vi "CustomPID_v3.0.vi"(0 "Kp":dbl=3e-05, 1 "Process Variable":dbl, 2 "Goal":dbl, 5 "Ki":dbl=5e-06, 7 "Kd":dbl=1e-06, 9 "N-Diff":i32=50, 11 "N-Int":i32=50, 12 "Reinit":bool, 13 "Max Ouput":dbl=1.0, 14 "Min Output":dbl=-1.0) -> (4 "Current Error":dbl, 8 "Command":dbl, 10 "Contribution Tracking":cluster{dbl, dbl, dbl}(graph), 15 "PID Tracking":cluster{"Goal Wheel Position":dbl, dbl}(graph)={"Goal Wheel Position"=0.0, -90.17571233858979})   [LabVIEW 2018]
uses:
  <vilib>/Analysis/NI_AALPro.lvlib
panel:
  out "Absolute Iterations":i32
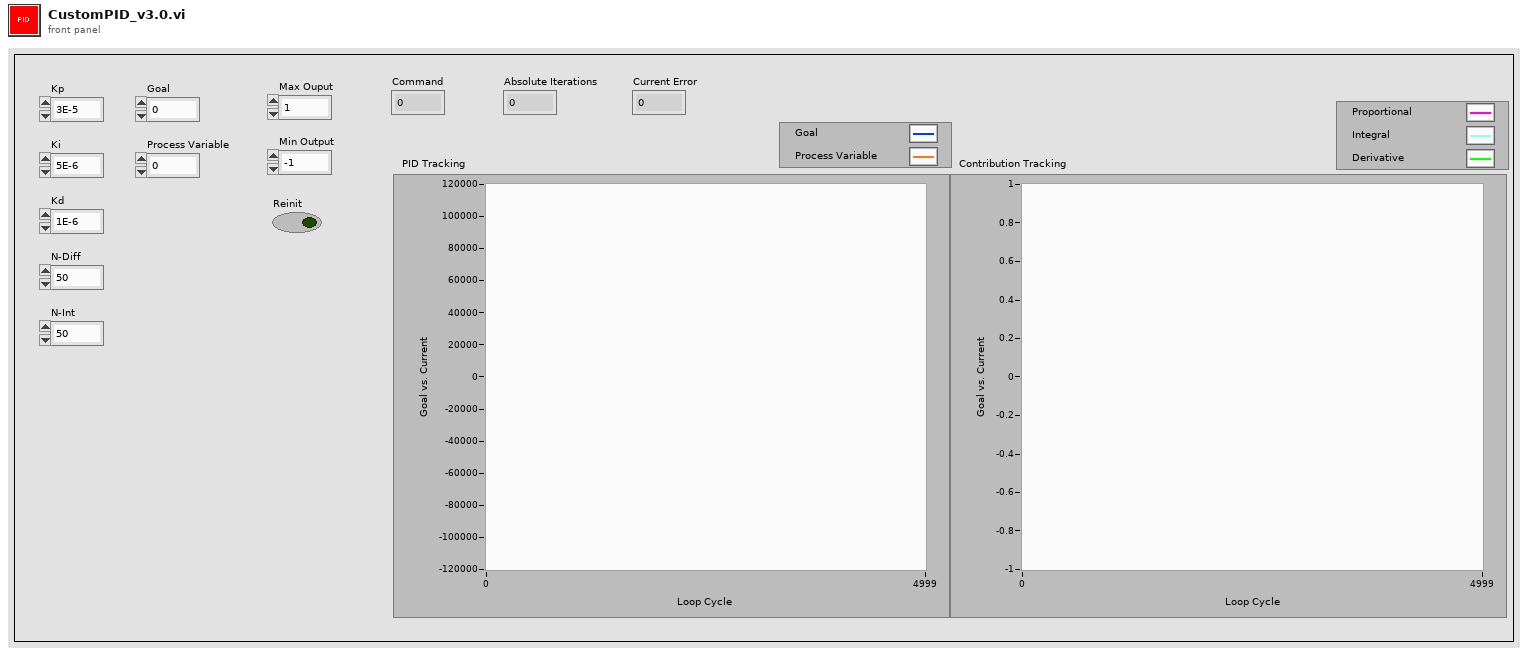
[diagram p1: front panel]
types:
  T1 = cluster{"Max Ouput":dbl, "Max Ouput":dbl, "Max Ouput":dbl}
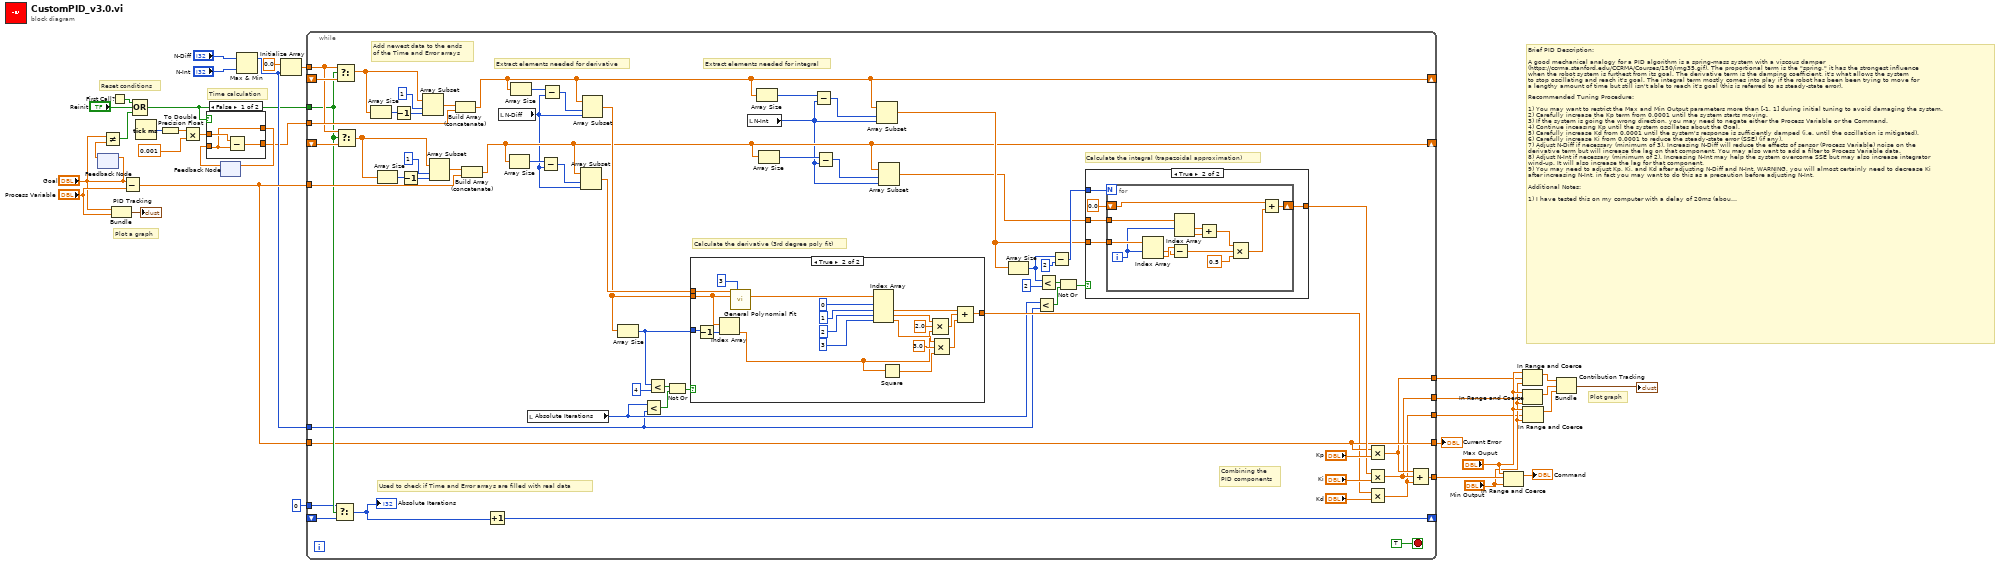
[diagram p0: block diagram]
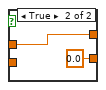
[diagram p2: hidden frame]
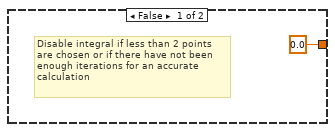
[diagram p3: hidden frame]
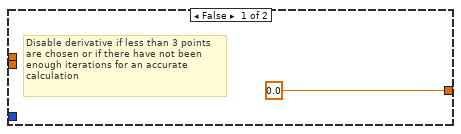
[diagram p4: hidden frame]
diagram:
  # "Plot graph"
  # "Time calculation"
  # "Brief PID Description:\n\nA good mechanical analogy for a PID algorithm is a spring-mass system with a viscous damper \n(https://ccrma.stanford.edu/CCRMA/Courses/150/img35.gif). The proportional term is the \"spring,\" it has the strongest influence\nwhen the robot system is furthest from its goal. The derivative term is the damping coefficient, it's what allows the system\nto stop oscillating and reach it's goal. The integral term mostly comes into play if the robot has been been trying to move for \na lengthy amount of time but still isn't able to reach it's goal (this is referred to as steady-state error).\n\nRecommended Tuning Procedure:\n\n1) You may want to restrict the Max and Min Output parameters more than [-1, 1] during initial tuning to avoid damaging the system.\n2) Carefully increase the Kp term from 0.0001 until the system starts moving.\n3) If the system is going the wrong direction, you may need to negate either the Process Variable or the Command.\n4) Continue inceasing Kp until the system oscillates about the Goal.\n5) Carefully increase Kd from 0.0001 until the system's response is sufficiently damped (i.e. until the oscillation is mitigated).\n6) Carefully increase Ki from 0.0001 to reduce the steady-state error (SSE) (if any).\n7) Adjust N-Diff if necessary (minimum of 3). Increasing N-Diff will reduce the effects of sensor (Process Variable) noise on the \nderivative term but will increase the lag on that component. You may also want to add a filter to Process Variable data.\n8) Adjust N-Int if necessary (minimum of 2). Increasing N-Int may help the system overcome SSE but may also increase integrator\nwind-up. It will also increase the lag for that component.\n9) You may need to adjust Kp, Ki, and Kd after adjusting N-Diff and N-Int. WARNING, you will almost certainly need to decrease Ki\nafter increasing N-Int, in fact you may want to do this as a precaution before adjusting N-Int. \n\nAdditional Notes:\n\n1) I have tested this on my computer with a delay of 20ms (about what I expect for the robot) and it appears to function correctly.\nThat being said I have NOT tested this on an actual, physical system. So exercise caution when testing it for the first time.\n2) Make sure that execution type for all instances of this VI are set to \"preallocated clone reentrant execution.\"\n3) Several parts of this VI were inspired by a PID algorithm written by Dr. Ira Hill at the University of Florida.\n4) If you have any questions, feel free to contact me at lrscime@ufl.edu."
  # "Plot a graph"
  # "Reset conditions"
  n1 = feedback-in #1("Goal") -> ()
  n2 = feedback #1() -> (w21:dbl)  [unwired: 1 in]
  n3 = Not Equal?(x="Goal", y=w21) -> (x != y?=w20:bool)
  n4 = First Call?() -> (First Call?: T/F=w29:bool)
  n5 = Bundle("Goal"="Goal", "Process Variable"="Process Variable") -> (→"PID Tracking":cluster{"Goal":dbl, "Process Variable":dbl})  [unwired: 1 in]
  n6 = Subtract(x="Goal", y="Process Variable") -> (x-y=w34:dbl)
  n7 = Compound Arithmetic op=OR(w29, "Reinit", w20) -> (w11:bool)
  n8 = Tick Count (ms)() -> (millisecond timer value=w18:u32)
  n9 = To Double Precision Float(number=w18) -> (double precision float=w17:dbl)
  n10 = Multiply(x=w17, y=0.001) -> (x*y=w15:dbl)
  n11 = feedback #2() -> (w13:dbl)  [unwired: 1 in]
  n12 = case shown="False" w11 {
    tunnel: w15 -> [w37 w39]
    tunnel: [w35 w39] -> w14
    tunnel: [w36 0.0] -> w12
    tunnel: w13 -> [w35 _]
    frame False {
      n13 = Subtract(x=w37, y=w35) -> (x-y=w36:dbl)
    }
    frame True {
    }
  }
  n14 = feedback-in #2(w14) -> ()
  n15 = Max & Min(x="N-Diff", y="N-Int") -> (max(x,y)=w23:i32)  [unwired: 1 out]
  n16 = Initialize Array(0.0 ("element"), w23) -> (w25:dbl[])
  n17 = while {
    tunnel: [w96] -> w31
    tunnel: w34 -> [w87]
    shift-right: [w75] -> _
    shift-left: _ -> [w61]
    tunnel: w12 -> [w91]
    shift-right: [w62] -> _
    shift-left: _ -> [w58]
    tunnel: w23 -> [w44]
    tunnel: w34 -> [w49]
    shift-right: [w68] -> _
    shift-left: _ -> [w55]
    tunnel: w11 -> [w54]
    tunnel: w25 -> [w59]
    tunnel: 0 -> [w50]
    tunnel: [w49] -> w10
    tunnel: [w42] -> w3
    tunnel: [w41] -> w2
    tunnel: [w40] -> w1
    stop <- TRUE stop-if-true
    # "Combining the\nPID components"
    # "Add newest data to the ends\nof the Time and Error arrays"
    # "Used to check if Time and Error arrays are filled with real data"
    # "Extract elements needed for integral"
    # "Extract elements needed for derivative"
    # "Calculate the integral (trapezoidal approximation)"
    # "Calculate the derivative (3rd degree poly fit)"
    n18 = Select(t=w50, s=w54, f=w55) -> (s? t:f=w56:i32)
    "Absolute Iterations" <- w56
    n19 = Select(t=w59, s=w54, f=w61) -> (s? t:f=w60:dbl[])
    n20 = Select(t=w59, s=w54, f=w58) -> (s? t:f=w57:dbl[])
    n21 = Array Size(array=w60) -> (size(s)=w94:i32)
    n22 = Array Size(array=w57) -> (size(s)=w89:i32)
    n23 = Decrement(x=w94) -> (x-1=w93:i32)
    n24 = Decrement(x=w89) -> (x-1=w88:i32)
    n25 = Array Subset(array=w60, index=1, length=w93) -> (w92:dbl[])
    n26 = Array Subset(array=w57, index=1, length=w88) -> (w86:dbl[])
    n27 = Build Array (concatenate)(w92, w91) -> (w75:dbl[])
    n28 = Build Array (concatenate)(w86, w87) -> (w62:dbl[])
    n29 = Increment(x=w56) -> (x+1=w68:i32)
    n30 = local read "N-Diff"() -> (w52:i32)
    n31 = Array Size(array=w62) -> (size(s)=w82:i32)
    n32 = Array Size(array=w75) -> (size(s)=w85:i32)
    n33 = local read "Absolute Iterations"() -> (w45:i32)
    n34 = Subtract(x=w82, y=w52) -> (x-y=w83:i32)
    n35 = Subtract(x=w85, y=w52) -> (x-y=w84:i32)
    n36 = Array Subset(array=w62, index=w83, length=w52) -> (w81:dbl[])
    n37 = Array Subset(array=w75, index=w84, length=w52) -> (w80:dbl[])
    n38 = Array Size(array=w80) -> (size(s)=w79:i32)
    n39 = Less?(x=w45, y=w44) -> (x < y?=w43:bool)
    n40 = Less?(x=w79, y=4) -> (x < y?=w47:bool)
    n41 = Not Or(1:w43, 2:w47) -> (0:w46:bool)
    n42 = case shown="True" w46 {
      tunnel: w81 -> [_ w136]
      tunnel: w79 -> [_ w135]
      tunnel: w80 -> [_ w133]
      tunnel: [0.0 w129] -> w48
      frame False {
        # "Disable derivative if less than 3 points \nare chosen or if there have not been \nenough iterations for an accurate \ncalculation"
      }
      frame True {
        n43 = Decrement(x=w135) -> (x-1=w134:i32)
        n44 = Index Array(array=w133, index=w134) -> (element=w122:dbl)
        n45 = call <vilib>:"General Polynomial Fit.vi"("Y"=w136, "polynomial order"=3, "X"=w133) -> ("Polynomial Coefficients"=w139:dbl[])  [unwired: 9 in, 3 out]
        n46 = Index Array(array=w139, index #1=0 ("index"), index #2=1 ("index"), index #3=2 ("index"), index #4=3 ("index")) -> (element #2=w128:dbl, element #3=w126:dbl, element #4=w123:dbl)  [unwired: 1 out]
        n47 = Square(x=w122) -> (x^2=w121:dbl)
        n48 = Compound Arithmetic op=MULTIPLY(w126, 2.0 ("y"), w122) -> (w127:dbl)
        n49 = Compound Arithmetic op=MULTIPLY(w123, 3.0 ("y"), w121) -> (w124:dbl)
        n50 = Compound Arithmetic op=ADD(w128, w127, w124) -> (w129:dbl)
      }
    }
    n51 = local read "N-Int"() -> (w51:i32)
    n52 = Array Size(array=w75) -> (size(s)=w77:i32)
    n53 = Array Size(array=w62) -> (size(s)=w74:i32)
    n54 = Subtract(x=w77, y=w51) -> (x-y=w76:i32)
    n55 = Subtract(x=w74, y=w51) -> (x-y=w73:i32)
    n56 = Array Subset(array=w75, index=w76, length=w51) -> (w63:dbl[])
    n57 = Array Subset(array=w62, index=w73, length=w51) -> (w53:dbl[])
    n58 = Array Size(array=w63) -> (size(s)=w66:i32)
    n59 = Less?(x=w45, y=w44) -> (x < y?=w70:bool)
    n60 = Less?(x=w66, y=2) -> (x < y?=w72:bool)
    n61 = Subtract(x=w66, y=2) -> (x-y=w65:i32)
    n62 = Not Or(1:w70, 2:w72) -> (0:w69:bool)
    n63 = case shown="True" w69 {
      tunnel: [0.0 w104] -> w67
      tunnel: w65 -> [_ w106]
      tunnel: w63 -> [_ w103]
      tunnel: w53 -> [_ w102]
      frame False {
        # "Disable integral if less than 2 points \nare chosen or if there have not been \nenough iterations for an accurate \ncalculation"
      }
      frame True {
        n64 = for {
          N: w106 -> [_]
          shift-right: [w118] -> w104
          shift-left: 0.0 -> [w119]
          tunnel: w103 -> [w117]
          tunnel: w102 -> [w110]
          i -> [w111]
          n65 = Index Array(array=w117, index #1=w111) -> (element #1=w115:dbl, element #2=w116:dbl)  [unwired: 1 in]
          n66 = Subtract(x=w116, y=w115) -> (x-y=w114:dbl)
          n67 = Index Array(array=w110, index #1=w111) -> (element #1=w108:dbl, element #2=w109:dbl)  [unwired: 1 in]
          n68 = Add(x=w108, y=w109) -> (x+y=w107:dbl)
          n69 = Compound Arithmetic op=MULTIPLY(w107, w114, 0.5 ("value")) -> (w112:dbl)
          n70 = Add(x=w119, y=w112) -> (x+y=w118:dbl)
        }
      }
    }
    n71 = Multiply(x=w49, y="Kp") -> (x*y=w42:dbl)
    n72 = Multiply(x=w67, y="Ki") -> (x*y=w41:dbl)
    n73 = Multiply(x=w48, y="Kd") -> (x*y=w40:dbl)
    n74 = Compound Arithmetic op=ADD(w42, w41, w40) -> (w96:dbl)
  }
  "Current Error" <- w10
  n75 = In Range and Coerce(upper limit="Max Ouput", x=w31, lower limit="Min Output") -> (coerced(x)=→"Command":dbl)  [unwired: 1 out]
  n76 = In Range and Coerce(upper limit="Max Ouput", x=w3, lower limit="Min Output") -> (coerced(x)=w8:dbl)  [unwired: 1 out]
  n77 = In Range and Coerce(upper limit="Max Ouput", x=w2, lower limit="Min Output") -> (coerced(x)=w7:dbl)  [unwired: 1 out]
  n78 = In Range and Coerce(upper limit="Max Ouput", x=w1, lower limit="Min Output") -> (coerced(x)=w6:dbl)  [unwired: 1 out]
  n79 = Bundle("Max Ouput"=w8, "Max Ouput"=w7, "Max Ouput"=w6) -> (→"Contribution Tracking":T1)  [unwired: 1 in]
